vi "Goodness_of_fit.vi"(6 "Weight":dbl[](array[numeric]), 8 "Wight=1":bool=TRUE, 9 "degree of freedom":i32=18, 10 "Best Fit":dbl[](array[numeric])=[2.5133927797533007, 2.0443196776808223, 1.6683862712863464, 1.3663985954311886, 1.1232146913577685, 0.9268754958096702, 0.767924086232023, 0.6388721880719148, 0.5337818538237559, 0.4479372491279151, 0.37758696419093674, 0.3197415484297478, 0.2720143071819939, 0.23249600792988317, 0.19965618068556185, 0.17226528849222822, 0.149333287300675, 0.13006106614617066, 0.11380201814502469, 0.10003158682935004, 0.0883230970064711, 0.07832854296592141, 0.06976329154982026, 0.06239388059369577], 11 "Y":dbl[](array[numeric])=[2.5134, 2.0443, 1.6684, 1.3664, 1.1232, 0.9269, 0.7679, 0.6389, 0.5338, 0.4479, 0.3776, 0.3197, 0.272, 0.2325, 0.1997, 0.1723, 0.1493, 0.1301, 0.1138, 0.1, 0.0883, 0.0783, 0.0698, 0.0624]) -> (1 "RMSE":dbl=2.9923229172110862e-05, 2 "R-square":dbl=0.9999999984855207, 3 "SSE":dbl=1.6117193593559995e-08)   [LabVIEW 2016]
uses:
  <vilib>/Analysis/baseanly.llb/Mean (DBL).vi
  <vilib>/Analysis/NI_AALBase.lvlib
panel:
  # "Goodness of fit"
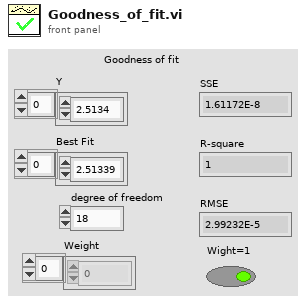
[diagram p1: front panel]
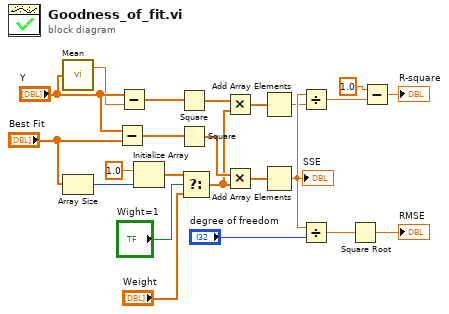
[diagram p0: block diagram]
diagram:
  n1 = call-poly <vilib>:"Mean.vi"("X"="Y") -> ("mean"=w18:dbl)  [unwired: 1 out]
  n2 = Array Size(array="Best Fit") -> (size(s)=w10:i32)
  n3 = Subtract(x="Y", y="Best Fit") -> (x-y=w23:dbl[])
  n4 = Subtract(x="Y", y=w18) -> (x-y=w12:dbl[])
  n5 = Initialize Array(1.0 ("element"), w10) -> (w8:dbl[])
  n6 = Square(x=w12) -> (x^2=w5:dbl[])
  n7 = Square(x=w23) -> (x^2=w3:dbl[])
  n8 = Select(t=w8, s="Wight=1", f="Weight") -> (s? t:f=w2:dbl[])
  n9 = Multiply(x=w5, y=w2) -> (x*y=w4:dbl[])
  n10 = Multiply(x=w3, y=w2) -> (x*y=w1:dbl[])
  n11 = Add Array Elements(numeric array=w4) -> (sum=w16:dbl)
  n12 = Add Array Elements(numeric array=w1) -> (sum=w17:dbl)
  "SSE" <- w17
  n13 = Divide(x=w17, y=w16) -> (x/y=w15:dbl)
  n14 = Divide(x=w17, y="degree of freedom") -> (x/y=w21:dbl)
  n15 = Square Root(x=w21) -> (sqrt(x)=→"RMSE":dbl)
  n16 = Subtract(x=1.0, y=w15) -> (x-y=→"R-square":dbl)
